vi "XY Variant to Persistent Data.vi"(8 "error in (no error)":errorcluster, 11 "Variant":variant) -> (0 "error out":errorcluster, 3 "Persistent Data":T1={"Label"="", "Graph Props"={"Plots"=[], "Legend:Number of Rows"=0, "Scale Properties"={"X.Auto"=FALSE, "X.Min"=0.0, "X.Max"=0.0, "X.IgnoreTS"=FALSE, "X.Precision"=0, "X.Label:"="", "X.LabelVis"=FALSE, "X.DefLabel"=FALSE, "Y.Auto"=FALSE, "Y.Min"=0.0, "Y.Max"=0.0, "Y.Format"=0, "Y.Precision:"=0, "Y.Label:"="", "Y.LabelVis"=FALSE, "Y.DefLabel"=FALSE, "X.Format"=0}, "Legend:Visible"=TRUE, "BgColor"=0, "Last Plot Width"=0, "Resize"=FALSE}, "UDP Data"={"Decimation"=0, "UDP Buffer Size"=0, "History Length"=0.0, "Update Rate"=enum."15 Hz", "Channel Paths"=[], "Channel Names"=[]}} {"Graph Props"."Scale Properties"."X.Format" items=["Decimal", "Scientific", "Engineering", "Binary", "Octal", "Hexadecimal", "Relative Time", "Time and Date", "SI", "Automatic"]; "Graph Props"."Scale Properties"."Y.Precision:" items=["0", "1", "2", "3", "4", "5", "6", "7"]; "Graph Props"."Scale Properties"."Y.Format" items=["Decimal", "Scientific", "Engineering", "Binary", "Octal", "Hexadecimal", "Relative Time", "Time and Date", "SI", "Automatic"]; "Graph Props"."Scale Properties"."X.Precision" items=["0", "1", "2", "3", "4", "5", "6", "7"]}, 5 "New":bool)   [LabVIEW 2012, in "Workspace MultiY Graph.lvlib"]
uses:
  Workspace MultiY Graph.lvlib
  XY Persistent Data.ctl
  XY Graph Properties.ctl
  XY Plot Properties.ctl
  XY Scale Properties.ctl
  XY Scale Precision.ctl
  XY Scale Format.ctl
  UDP Data.ctl
  Update Rate.ctl
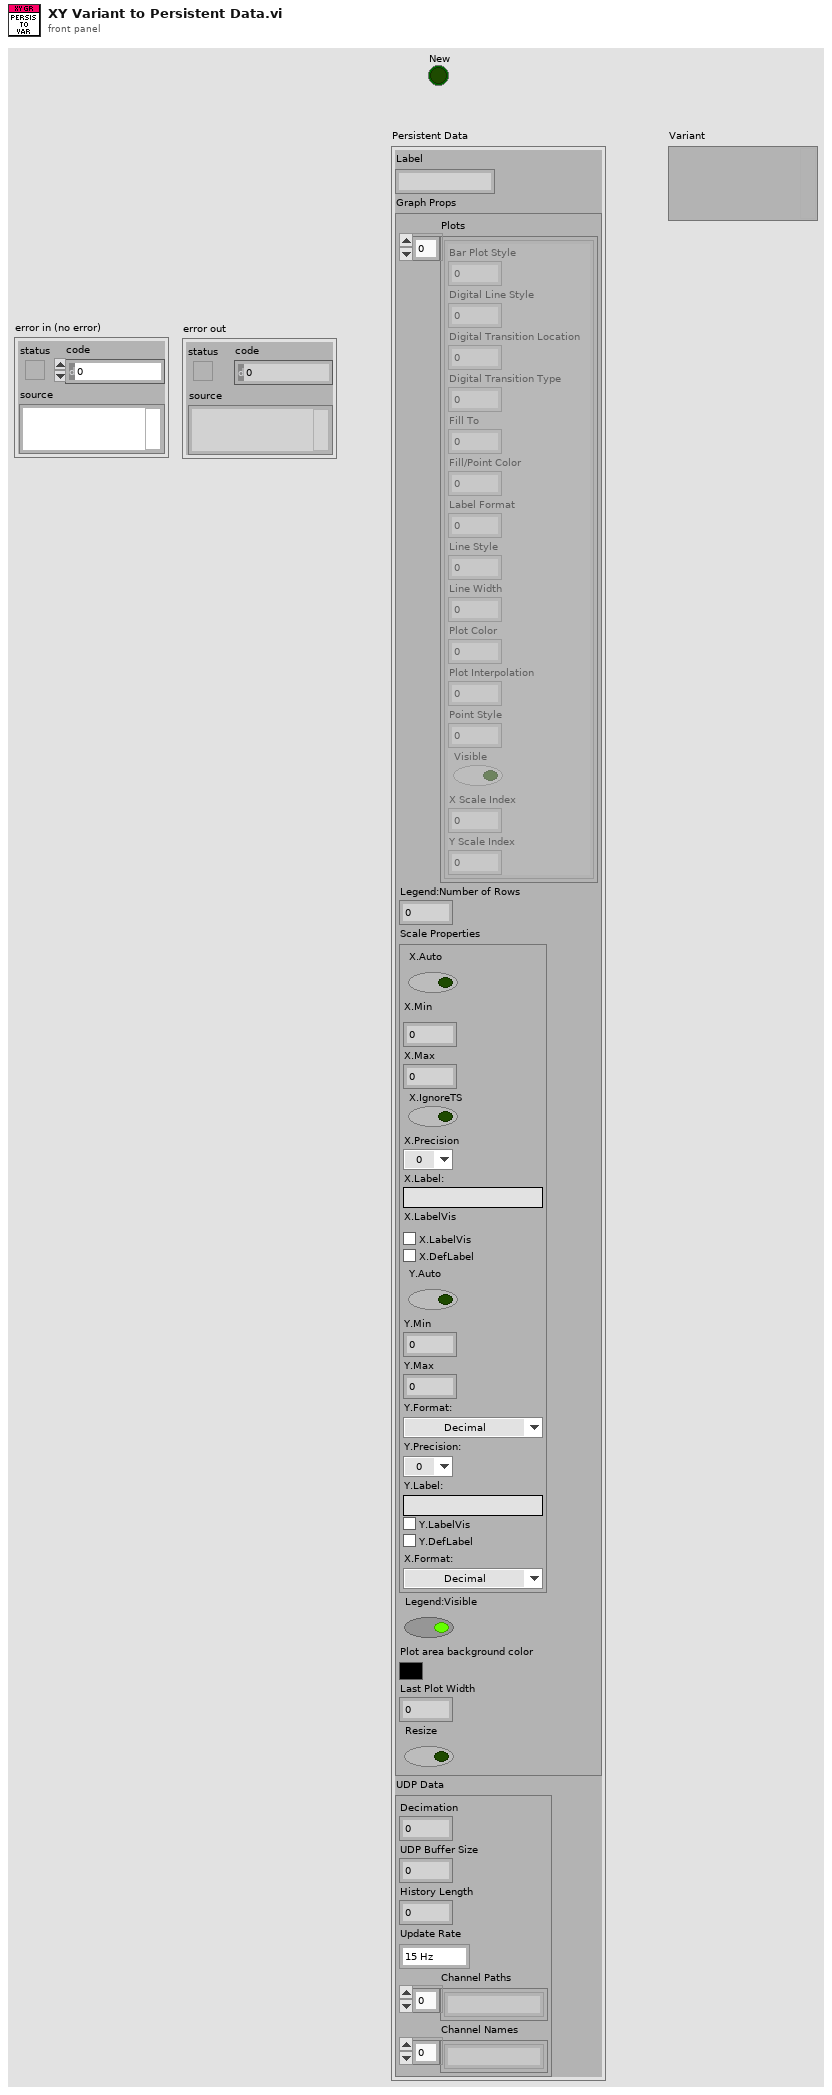
[diagram p1: front panel]
types:
  T1 = typedef "Workspace MultiY Graph.lvlib/XY Persistent Data.ctl" = cluster{"Label":string, "Graph Props":T2, "UDP Data":T7}
  T2 = typedef "Workspace MultiY Graph.lvlib/XY Graph Properties.ctl" = cluster{"Plots":T3[], "Legend:Number of Rows":u32, "Scale Properties":T4, "Legend:Visible":bool, "BgColor":u32, "Last Plot Width":u32, "Resize":bool}
  T3 = typedef "Workspace MultiY Graph.lvlib/XY Plot Properties.ctl" = cluster{"Bar Plot Style":u8, "Digital Line Style":u8, "Digital Transition Location":u8, "Digital Transition Type":u8, "Fill To":i16, "Fill/Point Color":u32, "Label Format":u8, "Line Style":u8, "Line Width":u8, "Plot Color":u32, "Plot Interpolation":u8, "Point Style":u8, "Visible":bool, "X Scale Index":u32, "Y Scale Index":u32}
  T4 = typedef "Workspace MultiY Graph.lvlib/XY Scale Properties.ctl" = cluster{"X.Auto":bool, "X.Min":dbl, "X.Max":dbl, "X.IgnoreTS":bool, "X.Precision":T5, "X.Label:":string, "X.LabelVis":bool, "X.DefLabel":bool, "Y.Auto":bool, "Y.Min":dbl, "Y.Max":dbl, "Y.Format":T6, "Y.Precision:":T5, "Y.Label:":string, "Y.LabelVis":bool, "Y.DefLabel":bool, "X.Format":T6}
  T5 = typedef "Workspace MultiY Graph.lvlib/XY Scale Precision.ctl" = u8
  T6 = typedef "Workspace MultiY Graph.lvlib/XY Scale Format.ctl" = u8
  T7 = typedef "Workspace MultiY Graph.lvlib/UDP Data.ctl" = cluster{"Decimation":i32, "UDP Buffer Size":u32, "History Length":dbl, "Update Rate":T8, "Channel Paths":string[], "Channel Names":string[]}
  T8 = typedef "Workspace MultiY Graph.lvlib/Update Rate.ctl" = enum8{"15 Hz", "10 Hz", "5 Hz", "4 Hz", "3 Hz", "2 Hz", "1 Hz", "0.5 Hz"}
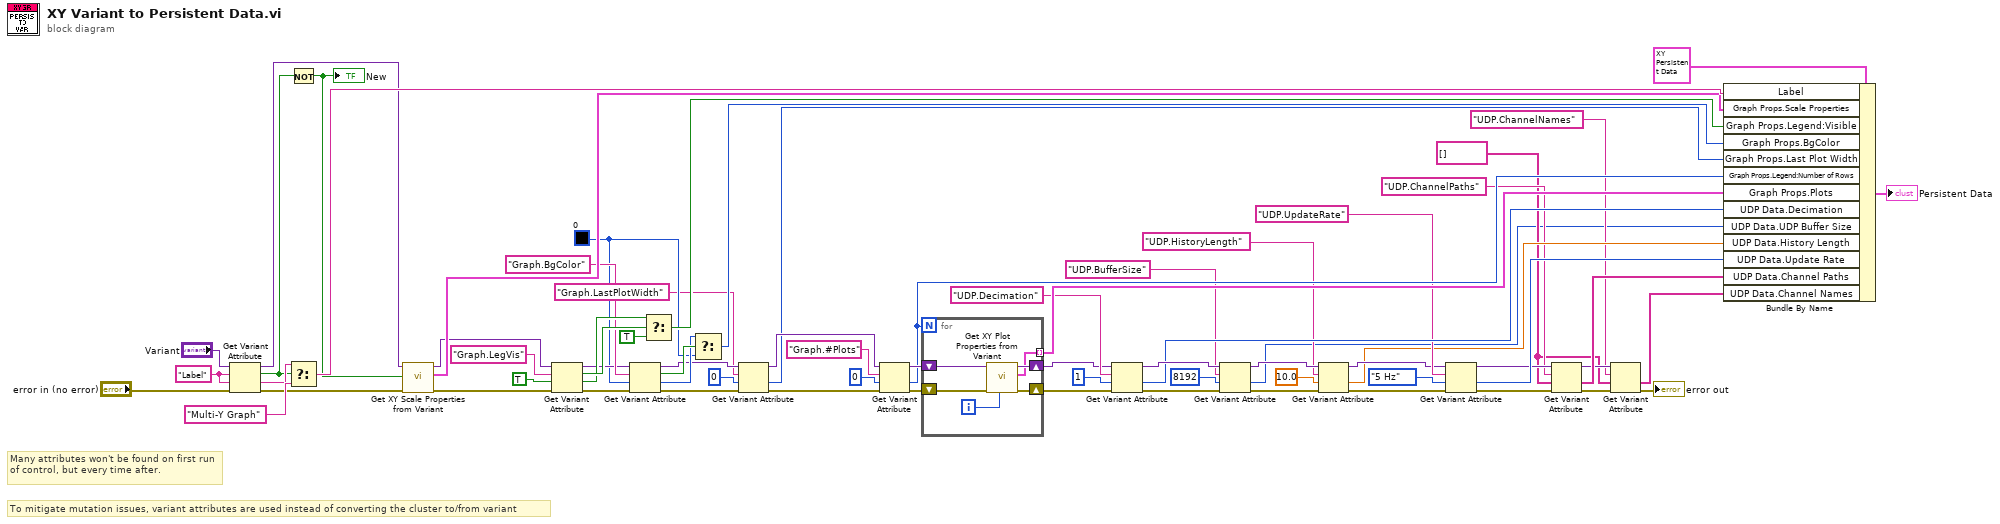
[diagram p0: block diagram]
diagram:
  w8 = string[] [] ("UDP Data.Channels")
  w40 = u32 0 ("BgColor")
  w68 = "Label" ("name")
  # "Many attributes won't be found on first run of control, but every time after."
  # "To mitigate mutation issues, variant attributes are used instead of converting the cluster to/from variant"
  n1 = Get Variant Attribute(Variant="Variant", name=w68, default value (empty Variant)=w68, error in="error in (no error)") -> (duplicate Variant=w56:variant, found=w38:bool, value=w58:string, error out=w57:errorcluster)
  n2 = Not(x=w38) -> (.not. x?=w37:bool)
  "New" <- w37
  n3 = Select(t=w58, s=w38, f="Multi-Y Graph" ("name")) -> (s? t:f=w60:string)
  n4 = call "Get XY Scale Properties from Variant.vi"("error in (no error)"=w57, "Use Defaults"=w37, "variant"=w56) -> ("error out"=w54:errorcluster, "Scale Properties"=w55:T4, "variant dup"=w53:variant)  [unwired: 6 in]
  n5 = Get Variant Attribute(Variant=w53, name="Graph.LegVis", default value (empty Variant)=TRUE, error in=w54) -> (duplicate Variant=w45:variant, found=w50:bool, value=w49:bool, error out=w44:errorcluster)
  n6 = Get Variant Attribute(Variant=w45, name="Graph.BgColor", default value (empty Variant)=w40, error in=w44) -> (duplicate Variant=w35:variant, found=w42:bool, value=w41:u32, error out=w43:errorcluster)
  n7 = Select(t=w49, s=w50, f=TRUE) -> (s? t:f=w48:bool)
  n8 = Select(t=w41, s=w42, f=w40) -> (s? t:f=w39:u32)
  n9 = Get Variant Attribute(Variant=w35, name="Graph.LastPlotWidth", default value (empty Variant)=u32 0 ("Graph Props.Last Plot Width"), error in=w43) -> (duplicate Variant=w34:variant, value=w31:u32, error out=w36:errorcluster)  [unwired: 1 out]
  n10 = Get Variant Attribute(Variant=w34, name="Graph.#Plots", default value (empty Variant)=u32 0 ("Graph Props.Legend:Number of Rows"), error in=w36) -> (duplicate Variant=w64:variant, value=w63:u32, error out=w65:errorcluster)  [unwired: 1 out]
  n11 = for {
    N: w63 -> [_]
    shift-right: [w76] -> w3
    shift-left: w64 -> [w77]
    shift-right: [w75] -> w2
    shift-left: w65 -> [w74]
    tunnel: [w72] -> w62 mode=indexing
    i -> [w73]
    n12 = call "Get XY Plot Properties from Variant.vi"("Plot#"=w73, "error in (no error)"=w74, "variant"=w77) -> ("error out"=w75:errorcluster, "Plot"=w72:T3, "variant dup"=w76:variant)  [unwired: 6 in]
  }
  n13 = Get Variant Attribute(Variant=w3, name="UDP.Decimation", default value (empty Variant)=1 ("UDP Data.Decimation"), error in=w2) -> (duplicate Variant=w28:variant, value=w27:i32, error out=w26:errorcluster)  [unwired: 1 out]
  n14 = Get Variant Attribute(Variant=w28, name="UDP.BufferSize", default value (empty Variant)=u32 8192 ("UDP Data.UDP Buffer Size"), error in=w26) -> (duplicate Variant=w23:variant, value=w1:u32, error out=w22:errorcluster)  [unwired: 1 out]
  n15 = Get Variant Attribute(Variant=w23, name="UDP.HistoryLength", default value (empty Variant)=10.0 ("UDP Data.History Length"), error in=w22) -> (duplicate Variant=w18:variant, value=w15:dbl, error out=w17:errorcluster)  [unwired: 1 out]
  n16 = Get Variant Attribute(Variant=w18, name="UDP.UpdateRate", default value (empty Variant)=Update_Rate."5 Hz" ("UDP Data.Update Rate"), error in=w17) -> (duplicate Variant=w13:variant, value=w14:T8, error out=w12:errorcluster)  [unwired: 1 out]
  n17 = Get Variant Attribute(Variant=w13, name="UDP.ChannelPaths", default value (empty Variant)=w8, error in=w12) -> (duplicate Variant=w9:variant, value=w10:string[], error out=w7:errorcluster)  [unwired: 1 out]
  n18 = Get Variant Attribute(Variant=w9, name="UDP.ChannelNames", default value (empty Variant)=w8, error in=w7) -> (value=w4:string[], error out=→"error out":errorcluster)  [unwired: 2 out]
  n19 = Bundle By Name(cluster=T1 {"Label"="", "Graph Props"={"Plots"=[], "Legend:Number of Rows"=0, "Scale Properties"={"X.Auto"=FALSE, "X.Min"=0.0, "X.Max"=0.0, "X.IgnoreTS"=FALSE, "X.Precision"=0, "X.Label:"="", "X.LabelVis"=FALSE, "X.DefLabel"=FALSE, "Y.Auto"=FALSE, "Y.Min"=0.0, "Y.Max"=0.0, "Y.Format"=0, "Y.Precision:"=0, "Y.Label:"="", "Y.LabelVis"=FALSE, "Y.DefLabel"=FALSE, "X.Format"=0}, "Legend:Visible"=FALSE, "BgColor"=0, "Last Plot Width"=0, "Resize"=FALSE}, "UDP Data"={"Decimation"=0, "UDP Buffer Size"=0, "History Length"=0.0, "Update Rate"=enum."15 Hz", "Channel Paths"=[], "Channel Names"=[]}} ("Persistent Data"), "Label"=w60, "Graph Props.Scale Properties"=w55, "Graph Props.Legend:Visible"=w48, "Graph Props.BgColor"=w39, "Graph Props.Last Plot Width"=w31, "Graph Props.Legend:Number of Rows"=w63, "Graph Props.Plots"=w62, "UDP Data.Decimation"=w27, "UDP Data.UDP Buffer Size"=w1, "UDP Data.History Length"=w15, "UDP Data.Update Rate"=w14, "UDP Data.Channel Paths"=w10, "UDP Data.Channel Names"=w4) -> (→"Persistent Data":T1)
